vi "Main DMA derived clock test.vi"() -> ()   [LabVIEW 2019]
uses:
  <vilib>/Platform/TimedLoop/XDataNode/timing_clust.ctl
  <vilib>/Platform/TimedLoop/XDataNode/nitl_modes.ctl
  <vilib>/Platform/TimedLoop/XDataNode/wakeup.ctl
  <vilib>/rvi/Emulation/niFpgaSctlEmulationGetInTimedLoop.vi
  <vilib>/rvi/Emulation/niFpgaProcessEmulError.vi
  <vilib>/rvi/Emulation/niFpgaEmulationReportErrorSimple.vi
  <vilib>/rvi/Emulation/niFpgaGetClockAttributes.vi
  <vilib>/rvi/Emulation/niFpgaCriticalErrorInLSC.vi
  <vilib>/rvi/eio/common/nirviEmuTemplateMethod_errors.vi
  <vilib>/rvi/interface/RandomDataEmulation/niFpgaRandomDataHandleErrors.vi
  <vilib>/platform/TimedLoop/XDataNode/XDataNode.xnode
  <vilib>/eio/EIONode/EIONode.xnode
  <vilib>/rvi/DataTransferAndStorage/Container/XNode/niFpgaContainer.xnode
  <vilib>/rvi/interface/RandomDataEmulation/nirviRandomDataFpgaReadWriteTemplate.vi
  <vilib>/Platform/TimedLoop/XDataNode/XDNodeRunTimeDep.lvlib
panel:
  in  "main_portlist_0":u16[](array[numeric])=[0, 0, 0, 0, 0, 0]
  out "port FIFO state":enum8{"reading", "waiting"}(ring)
  in  "xt end aux":u32
  in  "stop":bool
  out "GPIB counter":u16
  in  "GPIB0":u32
  in  "xt0":u32
  out "xt success":bool
  in  "xt end":u32
  in  "xt total":u32
  out "elapsed":u32
  out "xt counter":u32
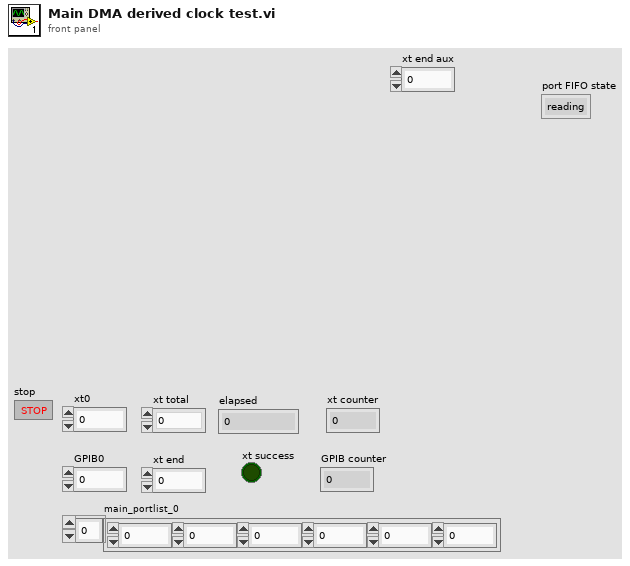
[diagram p1: front panel]
types:
  T1 = typedef "XDNodeRunTimeDep.lvlib/timing_clust.ctl" = cluster{"Expected End [f-1]":u64, "Actual End [f-1]":u64, "Finished Late? [f-1]":bool, "Expected End [i-1]":u64, "Actual End [i-1]":u64, "Finished Late? [i-1]":bool, "Expected Start [i]":u64, "Actual Start [i]":u64, "Expected Start [f]":u64, "Actual Start [f]":u64, "Source Name":string, "Structure Name":string, "Period":i64, "Deadline":i64, "Offset":i64, "Start":i64, "Priority":i32, "Timeout":i32, "Mode":T2, "Wakeup Reason":T3, "Error":errorcluster, "Source Type":string, "Secondary Source Type":string, "Global End Time":u64, "Global Start Time":u64, "Frame Duration":u64, "Iteration Duration":u64, "Assigned CPU":i32, "I/O Scan Engine Mode":u32}
  T2 = typedef "XDNodeRunTimeDep.lvlib/nitl_modes.ctl" = enum32{"No Change", "Process missed periods, maintain original phase", "Discard missed periods, maintain original phase", "Process missed periods, ignore original phase", "Discard missed periods, ignore original phase"}
  T3 = typedef "XDNodeRunTimeDep.lvlib/wakeup.ctl" = enum32{"Normal", "Aborted", "Asynchronous wakeup", "Timing source error", "Timed loop error", "Timeout"}
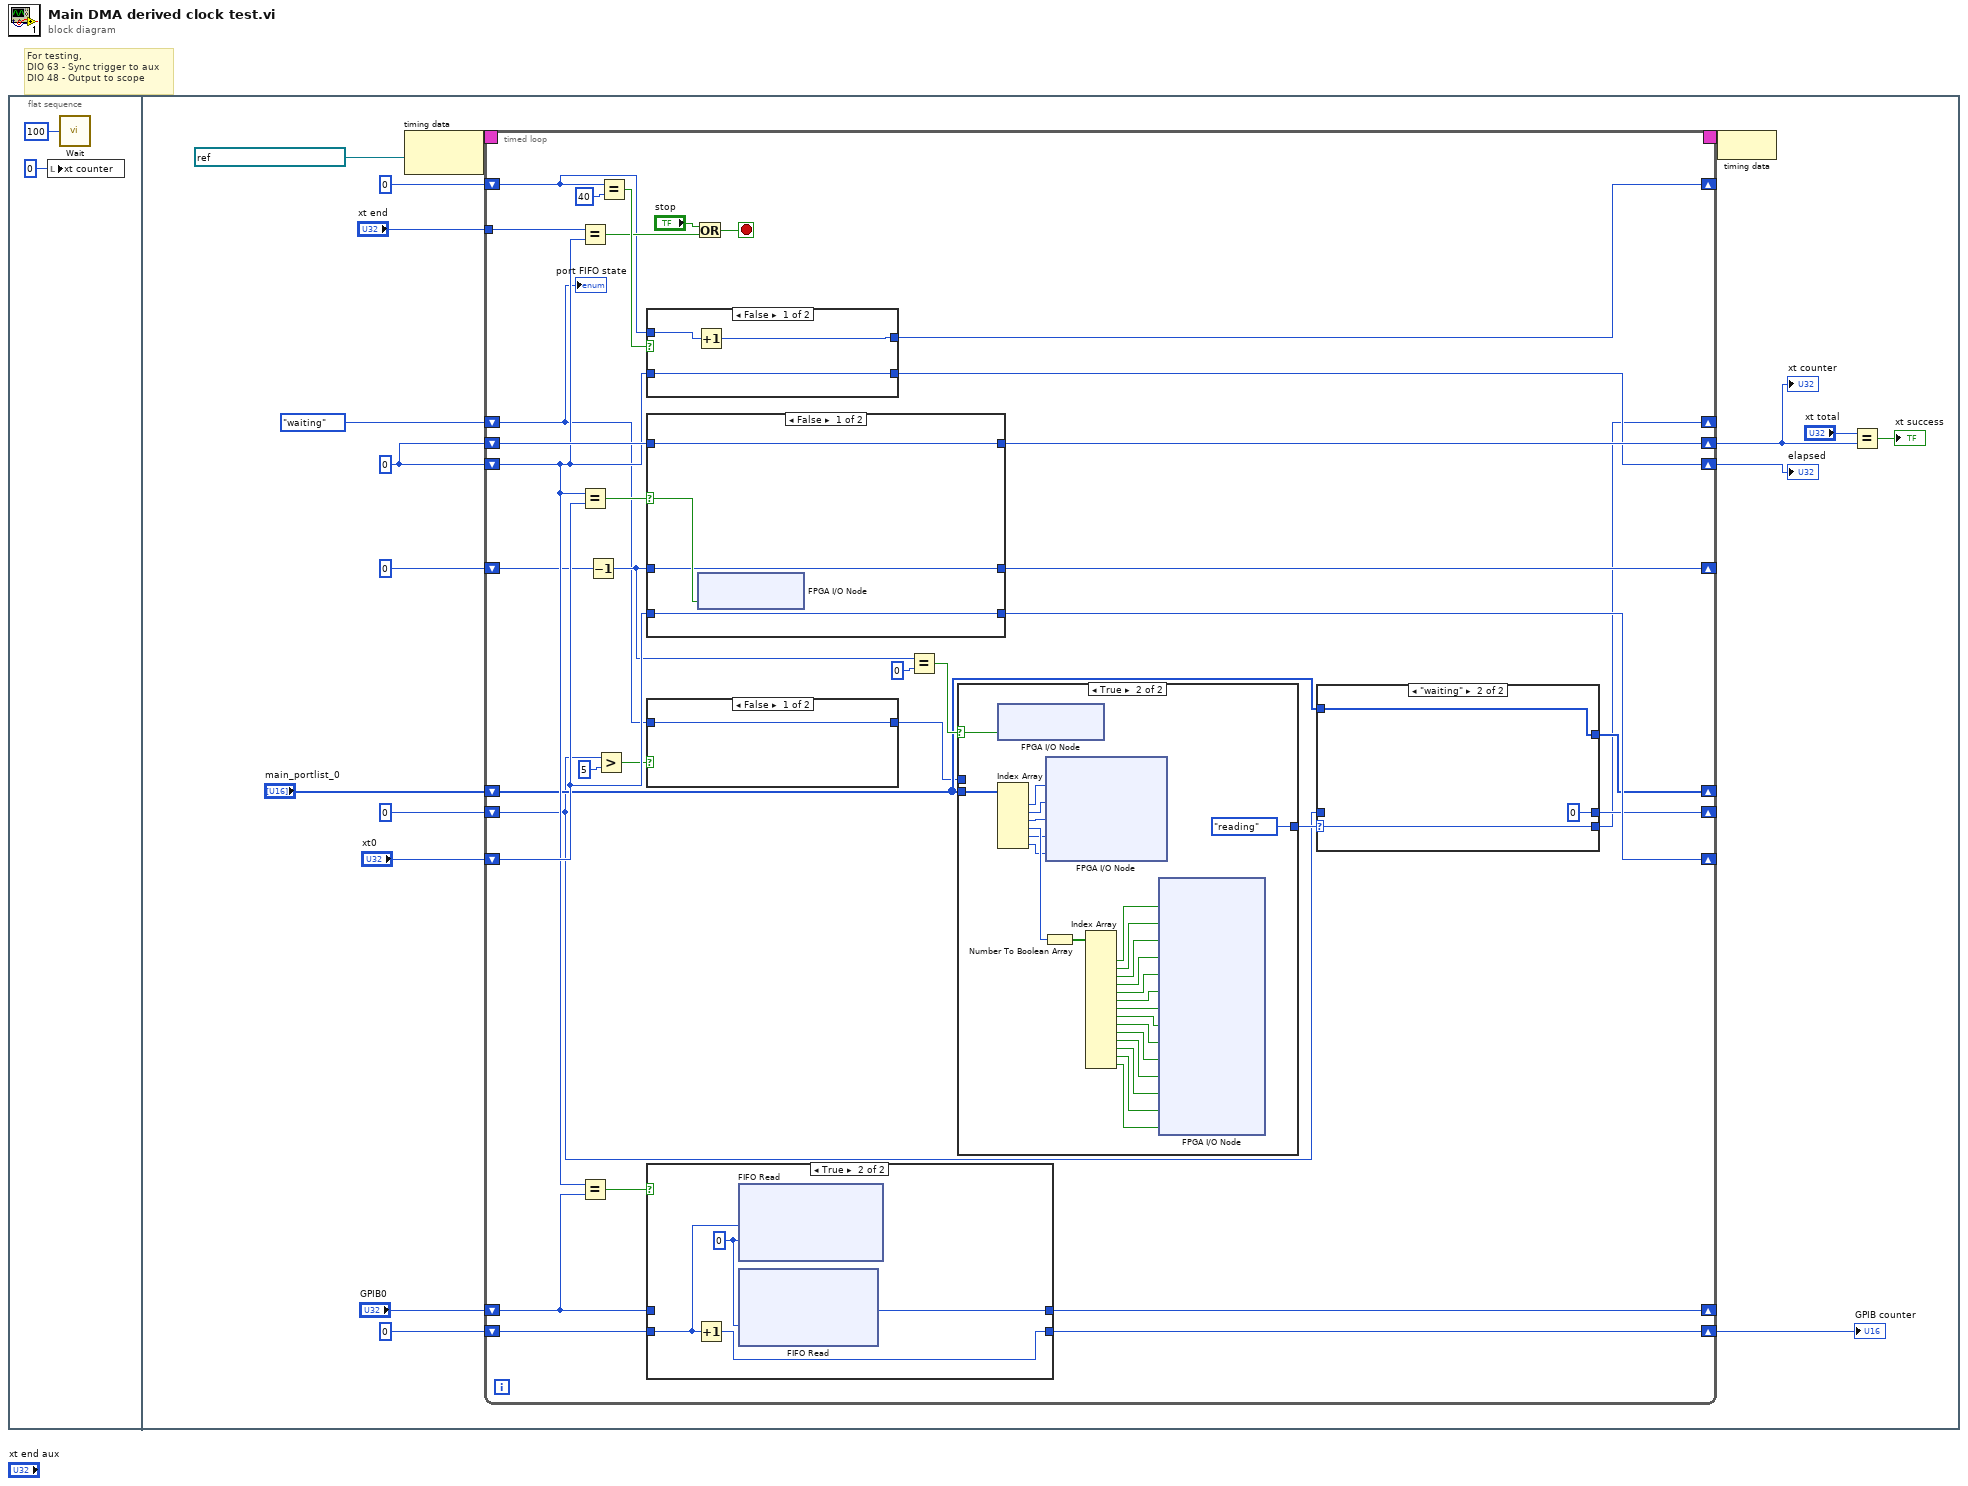
[diagram p0: block diagram]
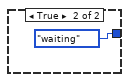
[diagram p2: hidden frame]
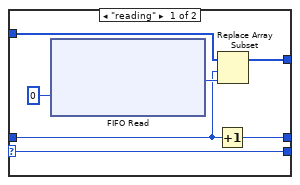
[diagram p3: hidden frame]
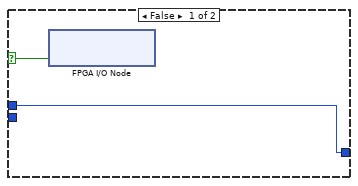
[diagram p4: hidden frame]
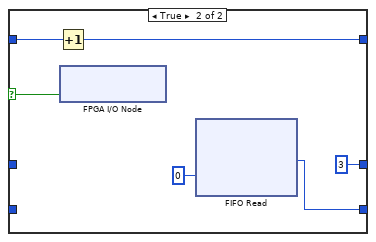
[diagram p6: hidden frame]
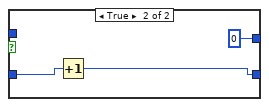
[diagram p7: hidden frame]
diagram:
  # "For testing,\nDIO 63 - Sync trigger to aux\nDIO 48 - Output to scope"
  n1 = flat-sequence {
    frame #0 {
      n2 = local write "xt counter"(u32 0 ("xt counter")) -> ()
      n3 = call "Wait"("Count(mSec)"=u8 100) -> ()  [unwired: 1 out]
    }
    frame #1 {
      w12 = u32 0
      n4 = node-c288(refnum<k21> "40 MHz Onboard Clock" ("Source Name")) -> (w18:T1)
      n5 = timed-loop {
        timing: w18 -> [_]
        timing-out: [_] -> w17
        shift-right: [w43] -> _
        shift-left: u8 0 -> [w38]
        shift-right: [w42] -> w10
        shift-left: w12 -> [w39]
        shift-right: [w54] -> _
        shift-left: "xt0" -> [w53]
        shift-right: [w49] -> _
        shift-left: "GPIB0" -> [w46]
        shift-right: [w51] -> w11
        shift-left: w12 -> [w52]
        shift-right: [w47] -> w8
        shift-left: u16 0 -> [w48]
        tunnel: "xt end" -> [w40]
        shift-right: [w33] -> _
        shift-left: 0 -> [w35]
        shift-right: [w21] -> _
        shift-left: enum8{"reading", "waiting"}."waiting" -> [w24]
        shift-right: [w22] -> _
        shift-left: u8 0 -> [w23]
        shift-right: [w29] -> _
        shift-left: "main_portlist_0" -> [w28]
        stop <- w45 stop-if-true
        n6 = Equal?(x=w40, y=w39) -> (x = y?=w41:bool)
        n7 = Equal?(x=w39, y=w53) -> (x = y?=w36:bool)
        n8 = Equal?(x=w39, y=w46) -> (x = y?=w50:bool)
        n9 = Decrement(x=w35) -> (x-1=w32:i32)
        n10 = Greater?(x=w23, y=u8 5) -> (0:w26:bool)
        n11 = Equal?(x=w38, y=u8 40) -> (x = y?=w55:bool)
        n12 = case shown="False" w55 {
          tunnel: w39 -> [w112 w115]
          tunnel: [w112 w114] -> w42
          tunnel: [w110 u8 0 ("y")] -> w43
          tunnel: w38 -> [w111 _]
          frame False {
            n13 = Increment(x=w111) -> (x+1=w110:u8)
          }
          frame True {
            n14 = Increment(x=w115) -> (x+1=w114:u32)
          }
        }
        n15 = case shown="False" w36 {
          selector: w36 -> [w101 w106]
          tunnel: [w103 w109] -> w54
          tunnel: w53 -> [w103 _]
          tunnel: w52 -> [w102 w108]
          tunnel: [w102 w107] -> w51
          tunnel: [w100 3] -> w33
          tunnel: w32 -> [w100 _]
          frame False {
            n16 = xnode "FPGA I/O Node"("RMC/DIO63"=w101) -> ()  [unwired: 1 in, 1 out]
          }
          frame True {
            n17 = Increment(x=w108) -> (x+1=w107:u32)
            n18 = xnode "FPGA I/O Node"("RMC/DIO63"=w106) -> ()  [unwired: 1 in, 1 out]
            n19 = xnode ("FIFO Read")("Timeout"=u8 0) -> ("Element"=w109:u32)  [unwired: 1 in, 2 out]
          }
        }
        n20 = case shown="False" w26 {
          tunnel: [w56 enum8{"reading", "waiting"}."waiting"] -> w25
          tunnel: w24 -> [w56 _]
          frame False {
          }
          frame True {
          }
        }
        n21 = case shown="True" w50 {
          tunnel: [w95 w99] -> w49
          tunnel: w48 -> [w94 w97]
          tunnel: [w94 w96] -> w47
          tunnel: w46 -> [w95 _]
          frame False {
          }
          frame True {
            w98 = u8 0 ("Timeout")
            n22 = Increment(x=w97) -> (x+1=w96:u16)
            n23 = xnode ("FIFO Read")("Element"=w97, "Timeout"=w98) -> ()  [unwired: 1 in, 2 out]
            n24 = xnode ("FIFO Read")("Timeout"=w98) -> ("Element"=w99:u32)  [unwired: 1 in, 2 out]
          }
        }
        n25 = Or(x="stop", y=w41) -> (x .or. y?=w45:bool)
        n26 = Equal?(x=w32, y=0 ("index")) -> (x = y?=w31:bool)
        n27 = case shown="True" w31 {
          selector: w31 -> [w69 w92]
          tunnel: [w68 enum8{"reading", "waiting"}."reading"] -> w30
          tunnel: w28 -> [_ w76]
          tunnel: w25 -> [w68 _]
          frame False {
            n28 = xnode "FPGA I/O Node"("RMC/DIO48"=w69) -> ()  [unwired: 1 in, 1 out]
          }
          frame True {
            n29 = xnode "FPGA I/O Node"("RMC/DIO48"=w92) -> ()  [unwired: 1 in, 1 out]
            n30 = Index Array(array=w76) -> (element #1=w75:u16, element #2=w74:u16, element #3=w73:u16, element #4=w72:u16, element #5=w71:u16, element #6=w70:u16)  [unwired: 6 in]
            n31 = Number To Boolean Array(number=w72) -> (Boolean array=w90:bool[])
            n32 = xnode "FPGA I/O Node"("RMC/DIO15:0"=w75, "RMC/DIO31:16"=w74, "RMC/DIO47:32"=w73, "RMC/DIO79:64"=w71, "RMC/DIO95:80"=w70) -> ()  [unwired: 5 in, 5 out]
            n33 = Index Array(array=w90) -> (element #2=w91:bool, element #3=w89:bool, element #4=w88:bool, element #5=w87:bool, element #6=w86:bool, element #7=w85:bool, element #8=w84:bool, element #9=w83:bool, element #10=w82:bool, element #11=w81:bool, element #12=w80:bool, element #13=w79:bool, element #14=w78:bool, element #15=w77:bool)  [unwired: 15 in, 1 out]
            n34 = xnode "FPGA I/O Node"("RMC/DIO49"=w91, "RMC/DIO50"=w89, "RMC/DIO51"=w88, "RMC/DIO52"=w87, "RMC/DIO53"=w86, "RMC/DIO54"=w85, "RMC/DIO55"=w84, "RMC/DIO56"=w83, "RMC/DIO57"=w82, "RMC/DIO58"=w81, "RMC/DIO59"=w80, "RMC/DIO60"=w79, "RMC/DIO61"=w78, "RMC/DIO62"=w77) -> ()  [unwired: 14 in, 14 out]
          }
        }
        n35 = case shown="\"waiting\"" w30 {
          selector: w30 -> [w58 w65]
          tunnel: [w64 w67] -> w29
          tunnel: w28 -> [w63 w67]
          tunnel: w23 -> [w60 _]
          tunnel: [w59 u8 0] -> w22
          tunnel: [w58 w65] -> w21
          frame "reading" {
            n36 = xnode ("FIFO Read")("Timeout"=0) -> ("Element"=w61:u16)  [unwired: 1 in, 2 out]
            n37 = Increment(x=w60) -> (x+1=w59:u8)
            n38 = Replace Array Subset(array=w63, new element=w61, index=w60) -> (w64:u16[])
          }
          frame "waiting" {
          }
        }
        "port FIFO state" <- w24
      }
      "elapsed" <- w10
      "xt counter" <- w11
      "GPIB counter" <- w8
      n39 = node-c288(w17) -> ()
      n40 = Equal?(x="xt total", y=w11) -> (x = y?=→"xt success":bool)
    }
  }
